vi "Pololu.Convert Value to Low and Hi Bytes.vi"(11 "Value":u16) -> (3 "Low_Hi Bytes":u8[](array[numeric]) format="%x")   [LabVIEW 2018, in "PololuCtrl.lvclass"]
uses:
  PololuCtrl.lvclass
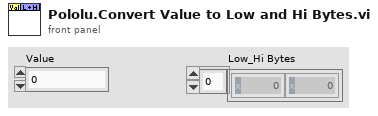
[diagram p1: front panel]
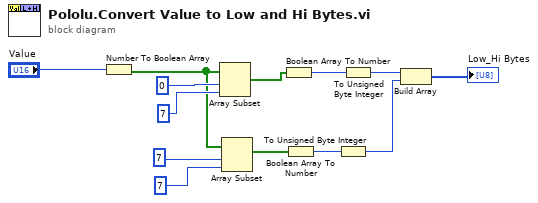
[diagram p0: block diagram]
diagram:
  n1 = Number To Boolean Array(number="Value") -> (Boolean array=w10:bool[])
  n2 = Array Subset(array=w10, index=0, length=7) -> (w7:bool[])
  n3 = Array Subset(array=w10, index=7, length=7) -> (w6:bool[])
  n4 = Boolean Array To Number(Boolean array=w7) -> (number=w5:u32)
  n5 = Boolean Array To Number(Boolean array=w6) -> (number=w4:u32)
  n6 = To Unsigned Byte Integer(number=w4) -> (unsigned 8bit integer=w2:u8)
  n7 = To Unsigned Byte Integer(number=w5) -> (unsigned 8bit integer=w3:u8)
  n8 = Build Array(w3, w2) -> (→"Low_Hi Bytes":u8[])
